vi "Load Properties.vi"(8 "error in":errorcluster caption="错误输入（无错误）", 10 "Properties":string[](array[string]), 11 "PanelRootNode 输入":refnum<class "PanelRootNode.lvclass"> caption="DNL_LabVIEW Object in") -> (0 "error out":errorcluster caption="错误输出", 3 "PanelRootNode 输出":refnum<class "PanelRootNode.lvclass"> caption="DNL_LabVIEW Object out")   [LabVIEW 2013, in "PanelRootNode.lvclass"]
uses:
  PanelRootNode.lvclass
  PanelDataNode/PanelDataNode.lvclass
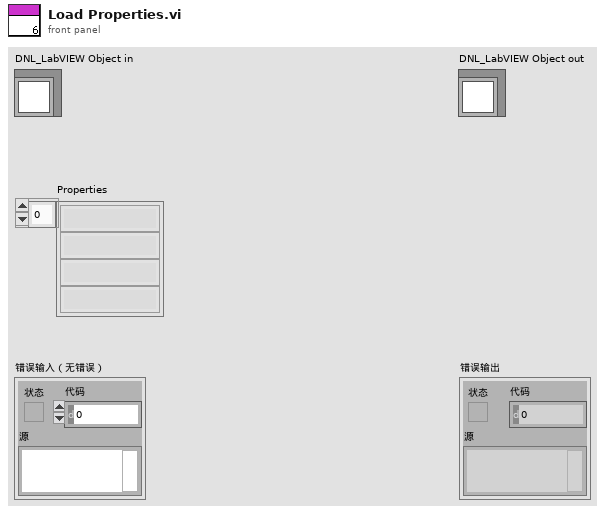
[diagram p1: front panel]
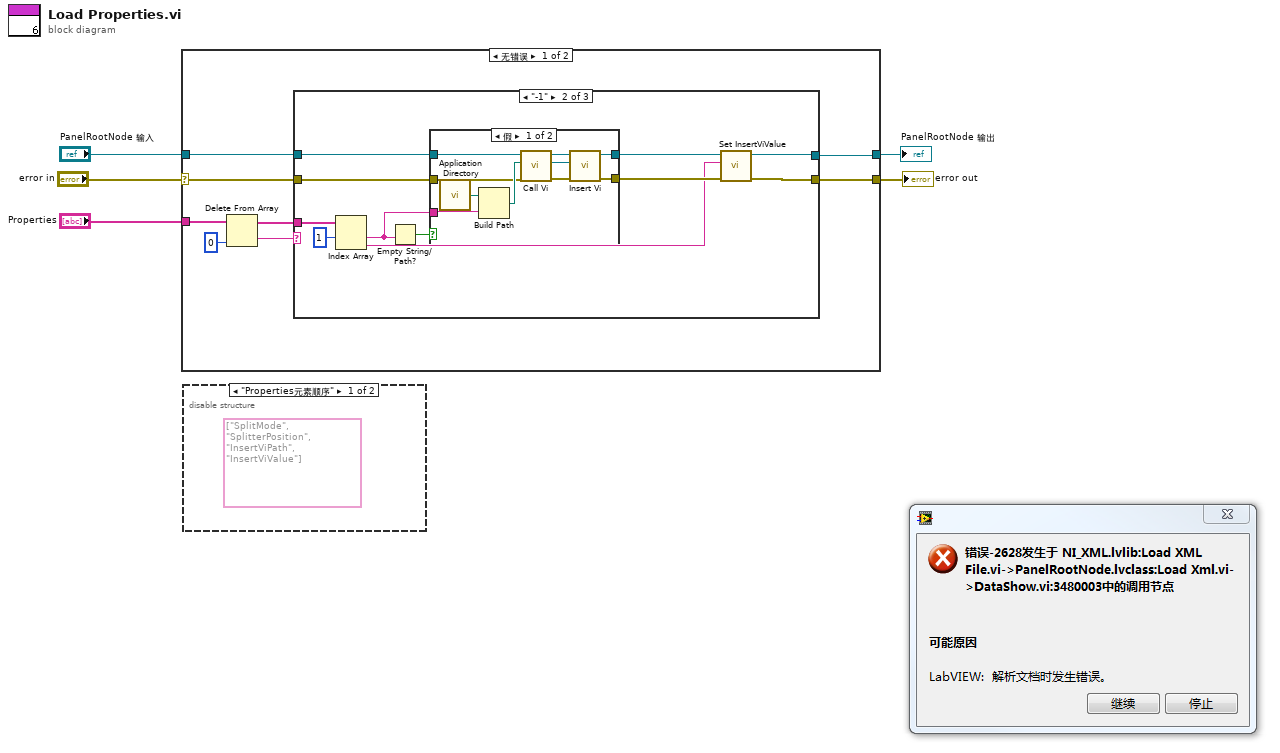
[diagram p0: block diagram]
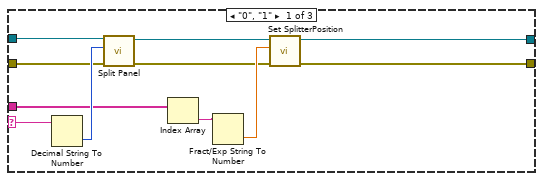
[diagram p3: hidden frame]
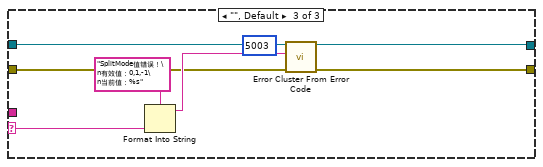
[diagram p5: hidden frame]
diagram:
  n1 = case shown="无错误" "error in" {
    selector: "error in" -> [w6 w56]
    tunnel: [w7 w56] -> w4
    tunnel: [w8 w55] -> w2
    tunnel: "PanelRootNode 输入" -> [w10 w55]
    tunnel: "Properties" -> [w13 _]
    frame No Error {
      n2 = Delete From Array(array=w13, index=0 ("索引")) -> (deleted portion=w9:string, array with subset deleted=w11:string[])  [unwired: 1 in]
      n3 = case shown="\"-1\"" w9 {
        selector: w9 -> [w24 _ w53]
        tunnel: w11 -> [w19 w35 _]
        tunnel: w10 -> [w23 w32 w54]
        tunnel: [w20 w29 w54] -> w8
        tunnel: [w15 w27 w50] -> w7
        tunnel: w6 -> [w14 w25 w49]
        frame "0", "1" {
          n4 = Decimal String To Number(string=w24) -> (number=w22:i32)  [unwired: 2 in, 1 out]
          n5 = call-dynamic "Split Panel.vi"("error in (no error)"=w14, "Split Mode"=w22, "PanelDataNode 输入"=w23) -> ("error out"=w16:errorcluster, "PanelDataNode 输出"=w21:refnum<class "PanelRootNode.lvclass">)  [unwired: 6 in, 1 out]
          n6 = Index Array(array=w19) -> (element=w18:string)  [unwired: 1 in]
          n7 = Fract/Exp String To Number(string=w18) -> (number=w17:dbl)  [unwired: 3 in, 1 out]
          n8 = call "Set SplitterPosition.vi"("error in (no error)"=w16, "Position(relative)"=w17, "PanelDataNode 输入"=w21) -> ("error out"=w15:errorcluster, "PanelDataNode 输出"=w20:refnum<class "PanelRootNode.lvclass">)  [unwired: 7 in]
        }
        frame "-1" {
          n9 = Index Array(array=w35, index #1=1 ("索引")) -> (element #1=w31:string, element #2=w26:string)  [unwired: 1 in]
          n10 = Empty String/Path?(string/path=w31) -> (empty?=w33:bool)
          n11 = case shown="假" w33 {
            tunnel: [w45 w47] -> w30
            tunnel: [w44 w46] -> w28
            tunnel: w31 -> [w42 _]
            tunnel: w32 -> [w41 w47]
            tunnel: w25 -> [w36 w46]
            frame False {
              n12 = call <vilib>:"Application Directory.vi"() -> ("Application Directory"=w43:path)
              n13 = Build Path(base path=w43, name or relative path=w42) -> (appended path=w39:path)
              n14 = call-dynamic "Call Vi.vi"("error in (no error)"=w36, "Vi Path"=w39, "PanelDataNode 输入"=w41) -> ("error out"=w37:errorcluster, "VI*"=w38:refnum<vi>, "PanelDataNode 输出"=w40:refnum<class "PanelRootNode.lvclass">)  [unwired: 6 in]
              n15 = call-dynamic "Insert Vi.vi"("error in (no error)"=w37, "VI*"=w38, "PanelDataNode 输入"=w40) -> ("error out"=w44:errorcluster, "PanelDataNode 输出"=w45:refnum<class "PanelRootNode.lvclass">)  [unwired: 7 in]
            }
            frame True {
            }
          }
          n16 = call-dynamic "Set InsertViValue.vi"("error in (no error)"=w28, "ViValue"=w26, "PanelDataNode 输入"=w30) -> ("error out"=w27:errorcluster, "PanelDataNode 输出"=w29:refnum<class "PanelRootNode.lvclass">)  [unwired: 7 in]
        }
        frame "", Default {
          n17 = Format Into String(format string="SplitMode值错误！\n有效值：0,1,-1\n当前值：%s" ("格式字符串"), w53) -> (resulting string=w51:string)  [unwired: 2 in, 1 out]
          n18 = call <vilib>:"Error Cluster From Error Code.vi"("error in (no error)"=w49, "error message (\"\")"=w51, "error code (0)"=5003) -> ("error out"=w50:errorcluster)  [unwired: 6 in]
        }
      }
    }
    frame Error {
    }
  }
  "error out" <- w4
  "PanelRootNode 输出" <- w2
  n19 = disable-structure shown="\"Properties元素顺序\"" {
    frame condition #0 {
      (unwired) string[] ["SplitMode", "SplitterPosition", "InsertViPath", "InsertViValue"]
    }
    frame condition #1 (active) {
    }
  }
